vi "valves_init.vi"(8 "error in (no error)":errorcluster, 11 "PortName":string="COM4") -> (0 "error out":errorcluster, 3 "reference out":refnum<k24>)   [LabVIEW 2018]
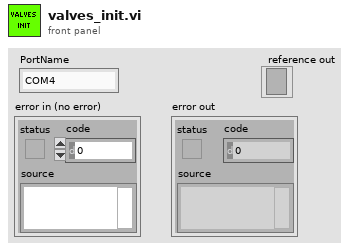
[diagram p1: front panel]
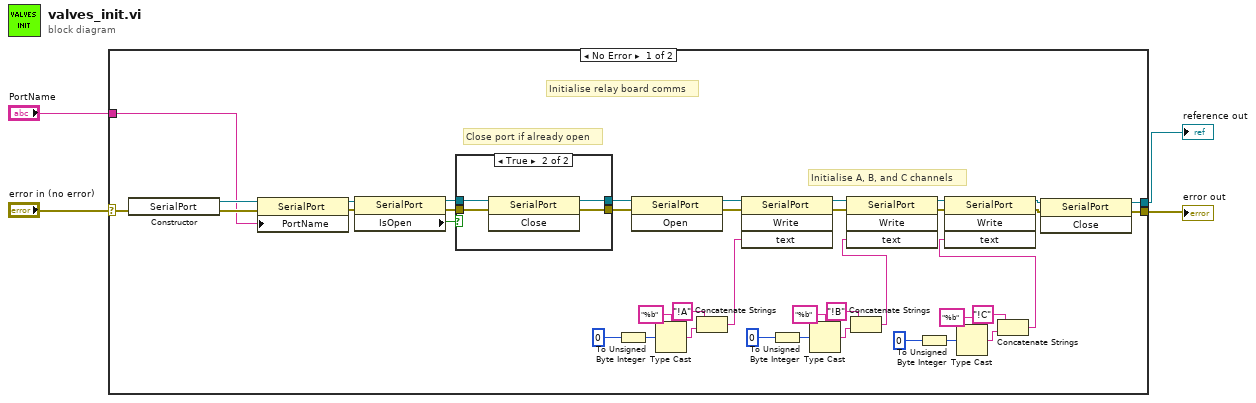
[diagram p0: block diagram]
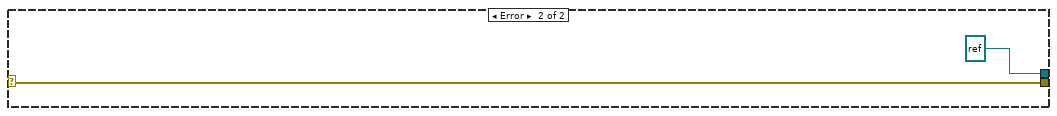
[diagram p3: hidden frame]
diagram:
  n1 = case shown="No Error" "error in (no error)" {
    selector: "error in (no error)" -> [w5 w50]
    tunnel: "PortName" -> [w34 _]
    tunnel: [w19 w50] -> w3
    tunnel: [w18 refnum<k24> refnum ("new reference")] -> w2
    frame No Error {
      # "Initialise relay board comms"
      # "Initialise A, B, and C channels"
      # "Close port if already open"
      n2 = constructor class="SerialPort"(error in=w5) -> (reference out=w40:refnum<k24>, error out=w41:errorcluster)  [unwired: 2 in, 1 out]
      n3 = property class="SerialPort"(reference=w40, error in=w41, "PortName"=w34) -> (reference out=w42:refnum<k24>, error out=w43:errorcluster)
      n4 = property class="SerialPort"(reference=w42, error in=w43) -> (reference out=w39:refnum<k24>, error out=w38:errorcluster, "IsOpen"=w37:bool)
      n5 = case shown="True" w37 {
        tunnel: [w44 w47] -> w36
        tunnel: [w45 w49] -> w35
        tunnel: w38 -> [w45 w46]
        tunnel: w39 -> [w44 w48]
        frame False {
        }
        frame True {
          n6 = invoke class="SerialPort" method="Close"(reference=w48, error in=w46) -> (reference out=w47:refnum<k24>, error out=w49:errorcluster)  [unwired: 1 in, 1 out]
        }
      }
      n7 = To Unsigned Byte Integer(number=u8 0) -> (unsigned 8bit integer=w28:u8)
      n8 = invoke class="SerialPort" method="Open"(reference=w36, error in=w35) -> (reference out=w26:refnum<k24>, error out=w27:errorcluster)  [unwired: 1 in, 1 out]
      n9 = Type Cast(type="%b", x=w28) -> (*(type *) &x=w30:string)
      n10 = Concatenate Strings("!A" ("string"), w30) -> (w33:string)
      n11 = invoke class="SerialPort" method="Write"(reference=w26, error in=w27, "text"=w33) -> (reference out=w25:refnum<k24>, error out=w24:errorcluster)  [unwired: 1 in, 2 out]
      n12 = To Unsigned Byte Integer(number=u8 0) -> (unsigned 8bit integer=w17:u8)
      n13 = Type Cast(type="%b", x=w17) -> (*(type *) &x=w15:string)
      n14 = Concatenate Strings("!B" ("string"), w15) -> (w7:string)
      n15 = invoke class="SerialPort" method="Write"(reference=w25, error in=w24, "text"=w7) -> (reference out=w23:refnum<k24>, error out=w22:errorcluster)  [unwired: 1 in, 2 out]
      n16 = To Unsigned Byte Integer(number=u8 0) -> (unsigned 8bit integer=w8:u8)
      n17 = Type Cast(type="%b", x=w8) -> (*(type *) &x=w10:string)
      n18 = Concatenate Strings("!C" ("string"), w10) -> (w6:string)
      n19 = invoke class="SerialPort" method="Write"(reference=w23, error in=w22, "text"=w6) -> (reference out=w21:refnum<k24>, error out=w20:errorcluster)  [unwired: 1 in, 2 out]
      n20 = invoke class="SerialPort" method="Close"(reference=w21, error in=w20) -> (reference out=w18:refnum<k24>, error out=w19:errorcluster)  [unwired: 1 in, 1 out]
    }
    frame Error {
    }
  }
  "error out" <- w3
  "reference out" <- w2
